vi "LVClass_CameraSet Set Parameter BoolValue.vi"(0 "CameraSet.lvclass":refnum<class "CameraSet.lvclass">, 5 "parameter_name":string, 7 "Value":bool, 11 "error in (no error)":errorcluster) -> (4 "CameraSet.lvclass":refnum<class "CameraSet.lvclass">, 15 "error out":errorcluster)   [LabVIEW 2020, in "CameraSet.lvclass"]
doc: "Camera parameter value setter for parameter of type boolean.\n\n<B>camera_setIn</B> : CameraSet object.\n<B>camera_setOut</B> : CameraSet object.\n<B>parameter_name</B> : Parameter name.\n<B>value</B> : Parameter value."
uses:
  CameraSet.lvclass
  CameraSet.lvclass/CameraSet.ctl
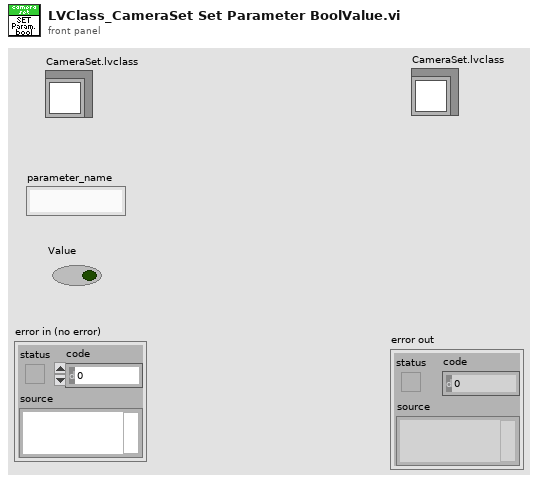
[diagram p1: front panel]
types:
  T1 = typedef "ClassID.ctl" = i64
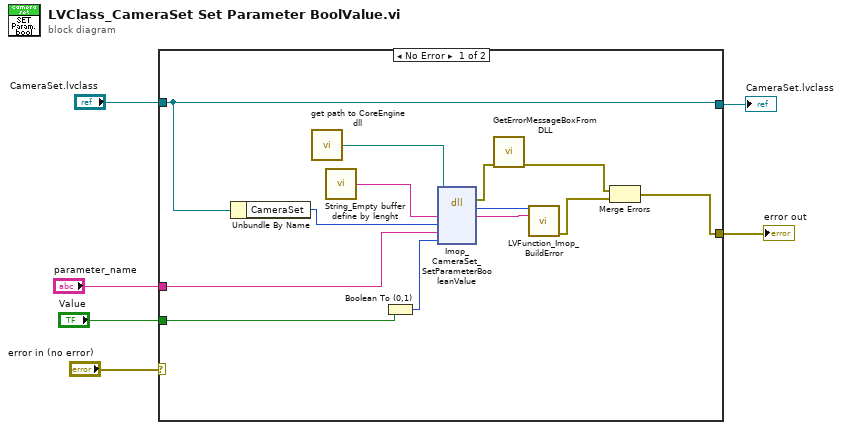
[diagram p0: block diagram]
diagram:
  n1 = case shown="No Error" "error in (no error)" {
    selector: "error in (no error)" -> [_ w20]
    tunnel: "CameraSet.lvclass" -> [w13 w21]
    tunnel: [w13 w21] -> w4
    tunnel: [w11 w20] -> w3
    tunnel: "Value" -> [w8 _]
    tunnel: "parameter_name" -> [w7 _]
    frame No Error {
      n2 = Unbundle By Name(w13) -> ("CameraSet"=w12:T1)
      n3 = call "get path to CoreEngine dll.vi"() -> ("path to wavekit library"=w16:path)  [unwired: 14 in, 1 out]
      n4 = call "String_Empty buffer define by lenght.vi"() -> ("Empty buffer"=w17:string)  [unwired: 1 in]
      n5 = Boolean To (0,1)(Boolean=w8) -> (0, 1=w14:i16)
      n6 = dll-call lib="D:/soft/HASO_v3/SVN_trunk/ImOpCoreEngine4_LV2011/DLLs/c_interface_vc100.dll" fn="Imop_CameraSet_SetParameterBooleanValue"(path in=w16, "message"=w17, "objet"=w12, "parameter_name"=w7, "value"=w14) -> (error out=w15:errorcluster, "return type"=w19:i32, "message"=w18:string)  [unwired: 5 in, 1 out]
      n7 = call "GetErrorMessageBoxFromDLL.vi"("error IN"=w15) -> ("error OUT"=w10:errorcluster)  [unwired: 10 in]
      n8 = call "LVFunction_Imop_BuildError.vi"("code"=w19, "String to Prepend to source (\"\")"=w18) -> ("error out"=w9:errorcluster)  [unwired: 13 in]
      n9 = Merge Errors(w10, w9) -> (w11:errorcluster)
    }
    frame Error {
    }
  }
  "CameraSet.lvclass" <- w4
  "error out" <- w3
